vi "Overwrite.vi"(10 "String":string, 11 "Value in":string) -> (3 "Value out":string)   [LabVIEW 2021]
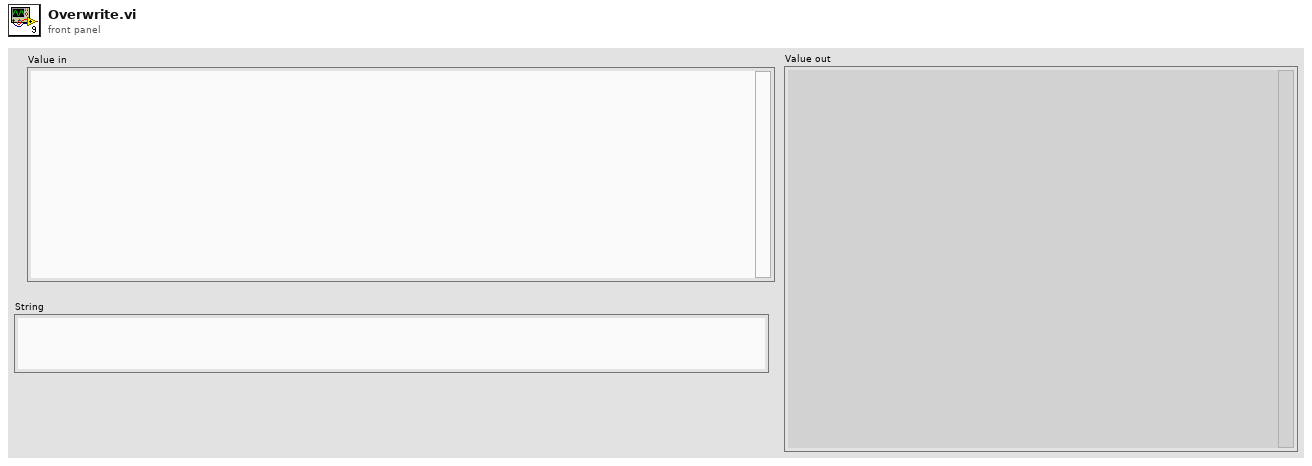
[diagram p1: front panel]
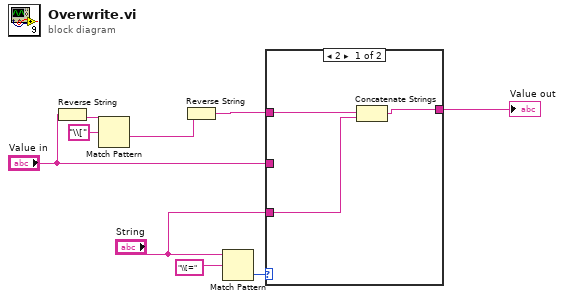
[diagram p0: block diagram]
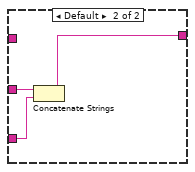
[diagram p2: hidden frame]
diagram:
  n1 = Reverse String(1:"Value in") -> (0:w8:string)
  n2 = Match Pattern(string=w8, regular expression="\\[") -> (after substring=w1:string)  [unwired: 1 in, 3 out]
  n3 = Reverse String(1:w1) -> (0:w9:string)
  n4 = Match Pattern(string="String", regular expression="\\[=") -> (offset past match=w5:i32)  [unwired: 1 in, 3 out]
  n5 = case shown="2" w5 {
    tunnel: w9 -> [w12 _]
    tunnel: "Value in" -> [_ w15]
    tunnel: "String" -> [w11 w14]
    tunnel: [w10 w13] -> w2
    frame 2 {
      n6 = Concatenate Strings(w12, w11) -> (w10:string)
    }
    frame Default {
      n7 = Concatenate Strings(w15, w14) -> (w13:string)
    }
  }
  "Value out" <- w2
